vi "Point Tool Histogram Results.vi"(1 "Connectivity":bool, 7 "Main_Gray Out":T1, 9 "ROI":T4, 11 "error in":errorcluster, 12 "Tolerance":sgl=20.0) -> (4 "Refnum out":T1, 6 "Statistics":T3, 10 "ROI Descriptor":T2 {"Contours"."Type" items=["No Selection", "Point", "Line", "Rectangle", "Oval", "Polygon", "Freehand Region", "Annulus", "Unused2", "Unused3", "Broken Line", "Freehand Line", "Rotated Rectangle"]}, 15 "error out":errorcluster)   [LabVIEW 2020]
uses:
  <vilib>/vision/Image Controls.llb/IMAQ Image.ctl
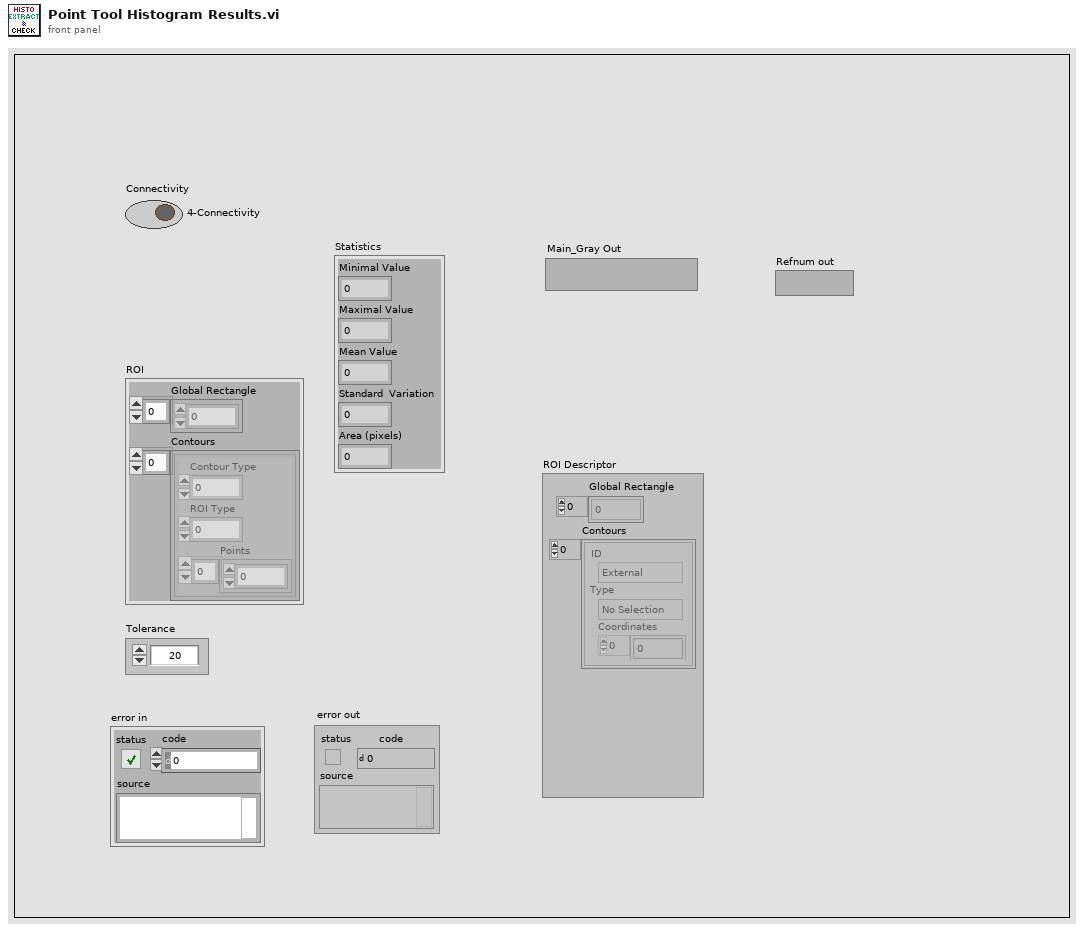
[diagram p1: front panel]
types:
  T1 = typedef "IMAQ Image.ctl" = refnum<image>
  T2 = typedef "ROI Descriptor" = cluster{"Global Rectangle":i32[], "Contours":cluster{"ID":enum32{"External", "Internal"}, "Type":u32, "Coordinates":i32[]}[]}
  T3 = cluster{"Minimal Value":sgl, "Maximal Value":sgl, "Mean Value":sgl, "Standard  Variation":sgl, "Area (pixels)":i32}
  T4 = cluster{"Global Rectangle":i32[], "Contours":cluster{"Contour Type":u32, "ROI Type":u32, "Points":i32[]}[]}
  T5 = cluster{"Contour Type":u32, "ROI Type":u32, "Points":i32[]}[]
  T6 = cluster{"Contour Type":u32, "ROI Type":u32, "Points":i32[]}
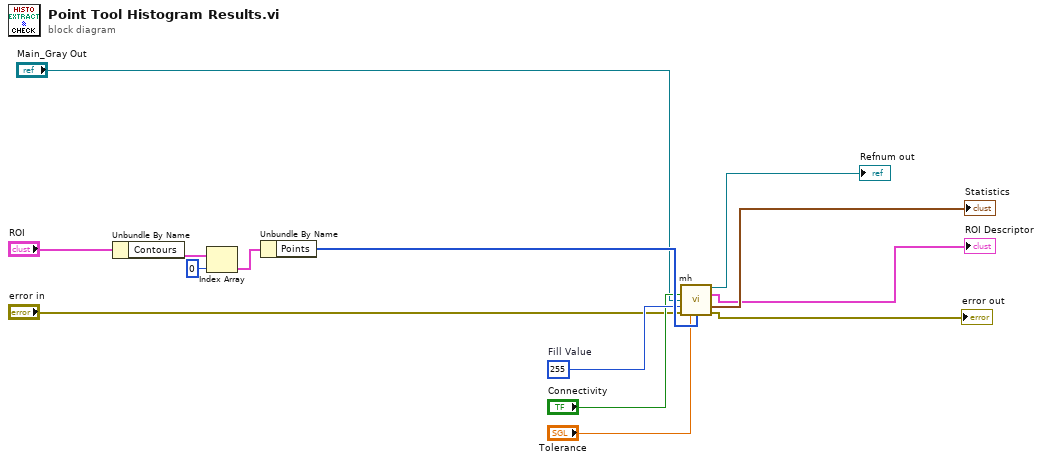
[diagram p0: block diagram]
diagram:
  w6 = u8 255  # Fill Value
  n1 = Unbundle By Name("ROI") -> ("Contours"=w12:T5)
  n2 = Index Array(array=w12, index=0) -> (element=w14:T6)
  n3 = Unbundle By Name(w14) -> ("Points"=w8:i32[])
  n4 = call "mh.vi"("Connectivity"="Connectivity", "Image Src"="Main_Gray Out", "Fill Value"=w6, "error in (no error)"="error in", "Tolerance"="Tolerance", "Hot spot (x,y)"=w8) -> ("Refnum out"=→"Refnum out":T1, "ROI Descriptor"=→"ROI Descriptor":T2, "Statistics"=→"Statistics":T3, "error out"=→"error out":errorcluster)  [unwired: 5 in, 1 out]
